vi "lfs_init.vi"(8 "error in (no error)":errorcluster) -> (0 "error out":errorcluster, 3 "lfs ref":refnum<class "IR sensor.lvclass">[](array[class]))   [LabVIEW 2019]
uses:
  FPGA_subVIs/low level/IR sensor/IR sensor.lvclass
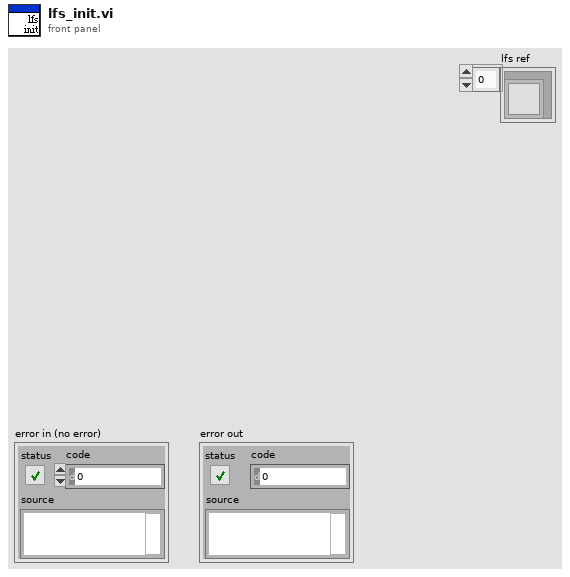
[diagram p1: front panel]
types:
  T1 = enum16{"IR.1", "IR.2", "IR.3", "IR.4", "IR.5", "IR.6", "IR.7", "IR.8"}
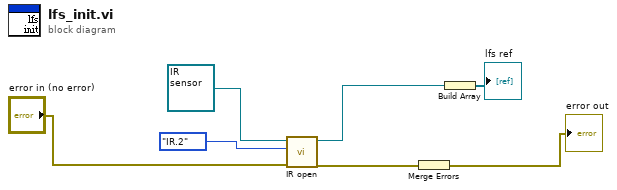
[diagram p0: block diagram]
diagram:
  n1 = call-dynamic "IR open.vi"("error in (no error)"="error in (no error)", "IR pin"=T1."IR.2", "IR sensor in"=refnum<class "IR sensor.lvclass"> refnum) -> ("error out"=w4:errorcluster, "IR sensor out"=w3:refnum<class "IR sensor.lvclass">)  [unwired: 7 in]
  n2 = Merge Errors(w4) -> (→"error out":errorcluster)
  n3 = Build Array(w3) -> (→"lfs ref":refnum<class "IR sensor.lvclass">[])
